vi "ErrorCluster.vi"() -> ()   [LabVIEW 2019]
panel:
  out "error out":errorcluster
  in  "String":string="My Name is Atul, My age is 29"
  in  "error in (no error)":errorcluster
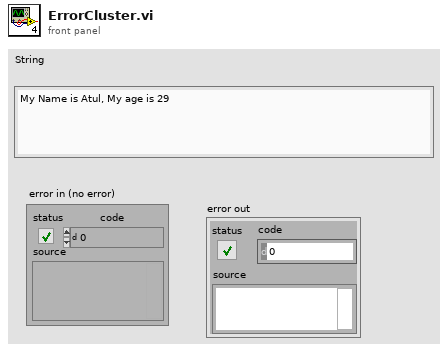
[diagram p1: front panel]
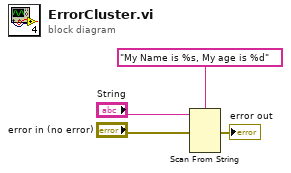
[diagram p0: block diagram]
diagram:
  n1 = Scan From String(format string="My Name is %s, My age is %d", input string="String", error in="error in (no error)") -> (error out=→"error out":errorcluster)  [unwired: 5 in, 2 out]
